vi "Clear Memory.vi"(8 "error in (no error)":errorcluster, 11 "VISA resource name":refnum<visa-resource-name>) -> (0 "error out":errorcluster, 3 "VISA resource name out":refnum<visa-resource-name>)   [LabVIEW 2014, in "Fluke 190 Series II.lvlib"]
doc: "Clears all saved setups, waveforms, and screens from internal memory.\n\n<b>Note:</b>\nThis command maybe not supported by several instruments."
uses:
  Fluke 190 Series II.lvlib
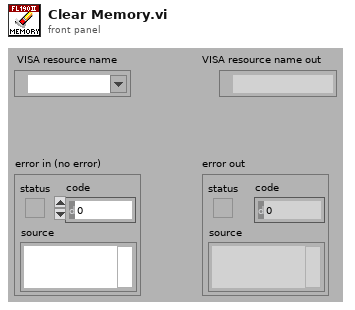
[diagram p1: front panel]
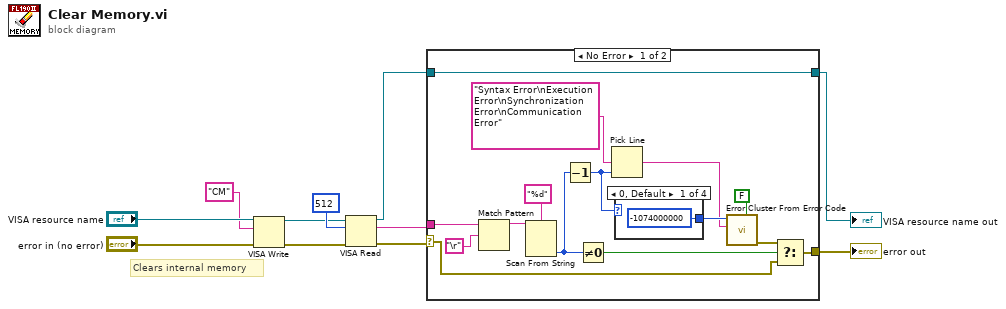
[diagram p0: block diagram]
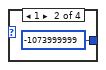
[diagram p2: hidden frame]
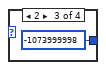
[diagram p3: hidden frame]
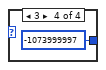
[diagram p4: hidden frame]
diagram:
  # "Clears internal memory"
  n1 = VISA Write(VISA resource name="VISA resource name", write buffer="CM", error in (no error)="error in (no error)") -> (VISA resource name out=w8:refnum<visa-resource-name>, error out=w7:errorcluster)  [unwired: 1 out]
  n2 = VISA Read(VISA resource name=w8, byte count=u32 512, error in (no error)=w7) -> (VISA resource name out=w5:refnum<visa-resource-name>, read buffer=w2:string, error out=w6:errorcluster)  [unwired: 1 out]
  n3 = case shown="No Error" w6 {
    selector: w6 -> [w21 w32]
    tunnel: w2 -> [w26 _]
    tunnel: w5 -> [w12 w31]
    tunnel: [w20 w32] -> w3
    tunnel: [w12 w31] -> w4
    frame No Error {
      n4 = Match Pattern(string=w26, regular expression="\r") -> (before substring=w24:string)  [unwired: 4 out]
      n5 = Scan From String(format string="%d", input string=w24) -> (output 1=w17:i32)  [unwired: 2 in, 4 out]
      n6 = Decrement(x=w17) -> (x-1=w15:i32)
      n7 = Not Equal To 0?(x=w17) -> (x != 0?=w22:bool)
      n8 = Pick Line(multi-line string="Syntax Error\nExecution Error\nSynchronization Error\nCommunication Error", line index=w15) -> (output string=w13:string)  [unwired: 1 out]
      n9 = case shown="0, Default" w15 {
        tunnel: [-1074000000 -1073999999 -1073999998 -1073999997] -> w14
        frame 0, Default {
        }
        frame 1 {
        }
        frame 2 {
        }
        frame 3 {
        }
      }
      n10 = call <vilib>:"Error Cluster From Error Code.vi"("is warning? (False)"=FALSE, "error message (\"\")"=w13, "error code (0)"=w14) -> ("error out"=w18:errorcluster)  [unwired: 2 in, 4 out]
      n11 = Select(t=w18, s=w22, f=w21) -> (s? t:f=w20:errorcluster)
    }
    frame Error {
    }
  }
  "VISA resource name out" <- w4
  "error out" <- w3
